vi "creae PID element from Object.vi"(11 "PID Loop in":refnum<class "PID Loop.lvclass">) -> (3 "line":T1)   [LabVIEW 2013, in "PID Module editor node.lvclass"]
uses:
  PID Module editor node.lvclass
  PID array element.ctl
  module/configuration/PID Loop.lvclass
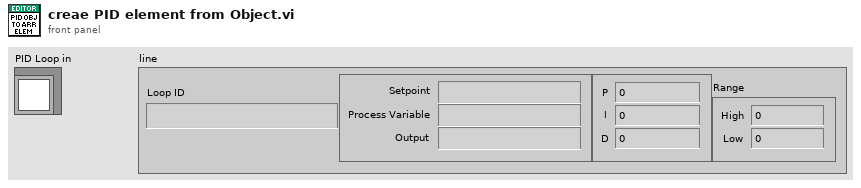
[diagram p1: front panel]
types:
  T1 = typedef "PID Module editor node.lvclass/PID array element.ctl" = cluster{"Loop ID":string, "Tags":cluster{"Setpoint":string, "Process Variable":string, "Output":string}, "Gains":cluster{"P":dbl, "I":dbl, "D":dbl}, "Range":cluster{"High":dbl, "Low":dbl}}
  T2 = typedef "PID Parameters.ctl" = cluster{"Setpoint Tag":string, "Process Variable Tag":string, "Output Tag":string}
  T3 = typedef "PID Gains.ctl" = cluster{"proportional gain (Kc)":dbl, "integral time (Ti, min)":dbl, "derivative time (Td, min)":dbl}
  T4 = typedef "PID Range.ctl" = cluster{"output high":dbl, "output low":dbl}
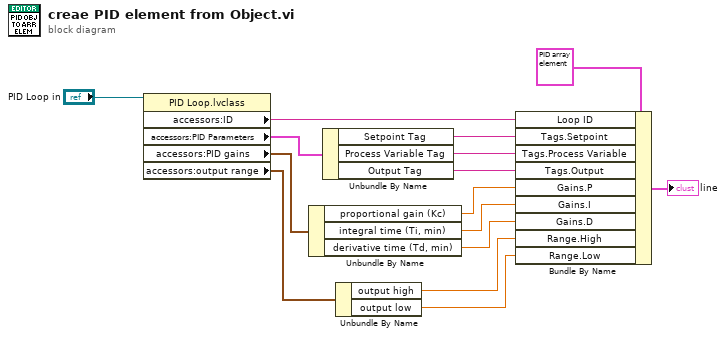
[diagram p0: block diagram]
diagram:
  n1 = property class="PID Loop.lvclass"(reference="PID Loop in") -> ("accessors:ID"=w15:string, "accessors:PID Parameters"=w3:T2, "accessors:PID gains"=w7:T3, "accessors:output range"=w11:T4)  [unwired: 1 in, 2 out]
  n2 = Unbundle By Name(w7) -> ("proportional gain (Kc)"=w8:dbl, "integral time (Ti, min)"=w9:dbl, "derivative time (Td, min)"=w10:dbl)
  n3 = Unbundle By Name(w3) -> ("Setpoint Tag"=w4:string, "Process Variable Tag"=w5:string, "Output Tag"=w6:string)
  n4 = Unbundle By Name(w11) -> ("output high"=w12:dbl, "output low"=w13:dbl)
  n5 = Bundle By Name(cluster=T1 {"Loop ID"="", "Tags"={"Setpoint"="", "Process Variable"="", "Output"=""}, "Gains"={"P"=1.0, "I"=0.01, "D"=0.0}, "Range"={"High"=100.0, "Low"=-100.0}} ("line"), "Loop ID"=w15, "Tags.Setpoint"=w4, "Tags.Process Variable"=w5, "Tags.Output"=w6, "Gains.P"=w8, "Gains.I"=w9, "Gains.D"=w10, "Range.High"=w12, "Range.Low"=w13) -> (→"line":T1)
